vi "DiffKinematics_toChassisSpeed.vi"(9 "RightVelocity":dbl, 10 "LeftVelocity":dbl, 11 "inDIFF_DRIVE_KINEMATICS":T1 {"TrackWidth_Meters" format="%20.4f"}) -> (3 "CHASSIS Speed":T2 {"vOmega" format="%10.3f"; "vY" format="%10.3f"; "vX" format="%10.3f"})   [LabVIEW 2019, in "Trajectory_Library.lvlib"]
doc: "Returns a chassis speed from left and right component velocities using forward kinematics.\n\nParameters:\n - in Diff Drive Kinematics -- This Differential Drive Kinematics data structure\n - LeftVelocity - The left wheel speed (meters/sec).\n - RightVelocity - The right wheel speed (meters/sec)\n\nReturns:\n - Chassis Speed - The chassis speed data structure"
uses:
  Trajectory_Library.lvlib
  TypeDef/CHASSIS_SPEEDS.ctl
  TypeDef/DIFF_DRIVE_KINEMATICS.ctl
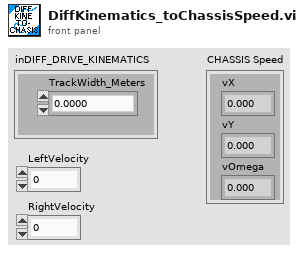
[diagram p1: front panel]
types:
  T1 = typedef "Trajectory_Library.lvlib/DIFF_DRIVE_KINEMATICS.ctl" = cluster{"TrackWidth_Meters":dbl}
  T2 = typedef "Trajectory_Library.lvlib/CHASSIS_SPEEDS.ctl" = cluster{"vX":dbl, "vY":dbl, "vOmega":dbl}
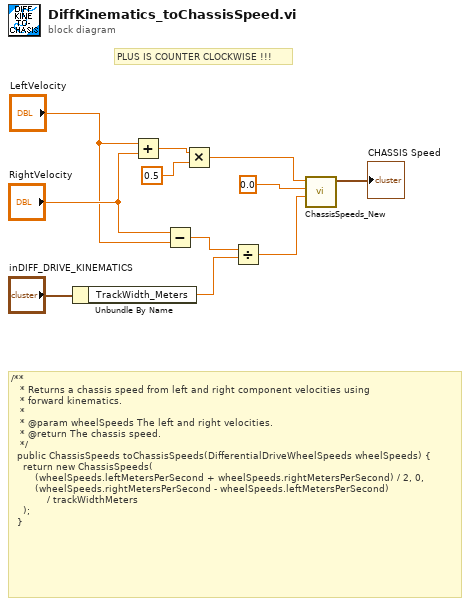
[diagram p0: block diagram]
diagram:
  # "PLUS IS COUNTER CLOCKWISE !!!"
  # "/**\n   * Returns a chassis speed from left and right component velocities using\n   * forward kinematics.\n   *\n   * @param wheelSpeeds The left and right velocities.\n   * @return The chassis speed.\n   */\n  public ChassisSpeeds toChassisSpeeds(DifferentialDriveWheelSpeeds wheelSpeeds) {\n    return new ChassisSpeeds(\n        (wheelSpeeds.leftMetersPerSecond + wheelSpeeds.rightMetersPerSecond) / 2, 0,\n        (wheelSpeeds.rightMetersPerSecond - wheelSpeeds.leftMetersPerSecond)\n            / trackWidthMeters\n    );\n  }"
  n1 = Unbundle By Name("inDIFF_DRIVE_KINEMATICS") -> ("TrackWidth_Meters"=w1:dbl)
  n2 = Add(x="LeftVelocity", y="RightVelocity") -> (x+y=w9:dbl)
  n3 = Subtract(x="RightVelocity", y="LeftVelocity") -> (x-y=w4:dbl)
  n4 = Multiply(x=w9, y=0.5) -> (x*y=w8:dbl)
  n5 = Divide(x=w4, y=w1) -> (x/y=w3:dbl)
  n6 = call "ChassisSpeeds_New.vi"("vAngular"=w3, "vY"=0.0, "vX"=w8) -> ("CHASSIS"=→"CHASSIS Speed":T2)  [unwired: 8 in]
